vi "9402_UI.vi"(8 "error in (no error)":errorcluster, 11 "Node Ptr":T1 format="%.0x") -> (0 "error out":errorcluster)   [LabVIEW 2020, in "Modules.lvlib" / "9402.lvclass"]
uses:
  9402.lvclass
  <vilib>/NI VeriStand/Custom Device API/Custom Device Item Ref.ctl
  RSI Module/SubPanel Command.ctl
  C:/Users/nitest/Desktop/Git 2020/niveristand-scan-engine-module-libraries/Source/RSI Module/RSI Module.lvclass
  9402.lvclass/9402.ctl
  RSI Module/RSI Module.lvclass
  <vilib>/NI VeriStand/Custom Device API/Custom Device API.lvlib
panel:
  in  "_Channels":u32[](array[ring]) items=["Input", "Output"]
  out "_Selected Channel(s) Settings Label":string="Selected Channel(s) Settings"
  in  "Channels":i32[](listbox)
  in  "LineDirectionVal":u32(ring) caption="Direction" items=["Input", "Output"]
  in  "SubPanel Event":refnum<user-event>
  in  "Header":cluster{"Section Name":string}={"Section Name"="NI 9205 Settings"}
  in  "BadLineDirectionVal":u32(ring) caption="Direction" items=["Input", "Output", "X"]
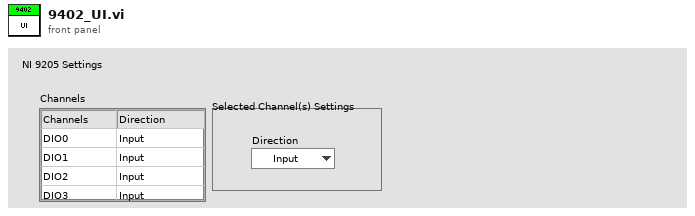
[diagram p1: front panel]
types:
  T1 = typedef "Custom Device API.lvlib/Custom Device Item Ref.ctl" = u64
  T2 = typedef "Modules.lvlib/RSI Module.lvclass/Module Models.ctl" = enum16{"Empty", "NI 9201", "NI 9203", "NI 9205", "NI 9206", "NI 9207", "NI 9208", "NI 9209", "NI 9210", "NI 9211", "NI 9212", "NI 9213", "NI 9214", "NI 9215", "NI 9216", "NI 9217", "NI 9219", "NI 9220", "NI 9221", "NI 9222", "NI 9223", "NI 9224", "NI 9225", "NI 9226", "NI 9227", "NI 9228", "NI 9229", "NI 9233", "NI 9234", "NI 9235", "NI 9236", "NI 9237", "NI 9239", "NI 9242", "NI 9244", "NI 9253", "NI 9263", "NI 9264", "NI 9265", "NI 9266", "NI 9269", "NI 9344", "NI 9350", "NI 9375", "NI 9401", "NI 9402", "NI 9403", "NI 9411", "NI 9421", "NI 9422", "NI 9423", "NI 9425", "NI 9426", "NI 9435", "NI 9436", "NI 9437", "NI 9472", "NI 9474", "NI 9475", "NI 9476", "NI 9477", "NI 9478", "NI 9481", "NI 9482", "NI 9485"}
  T3 = typedef "Modules.lvlib/RSI Module.lvclass/SubPanel Command.ctl" = enum16{"Stop"}
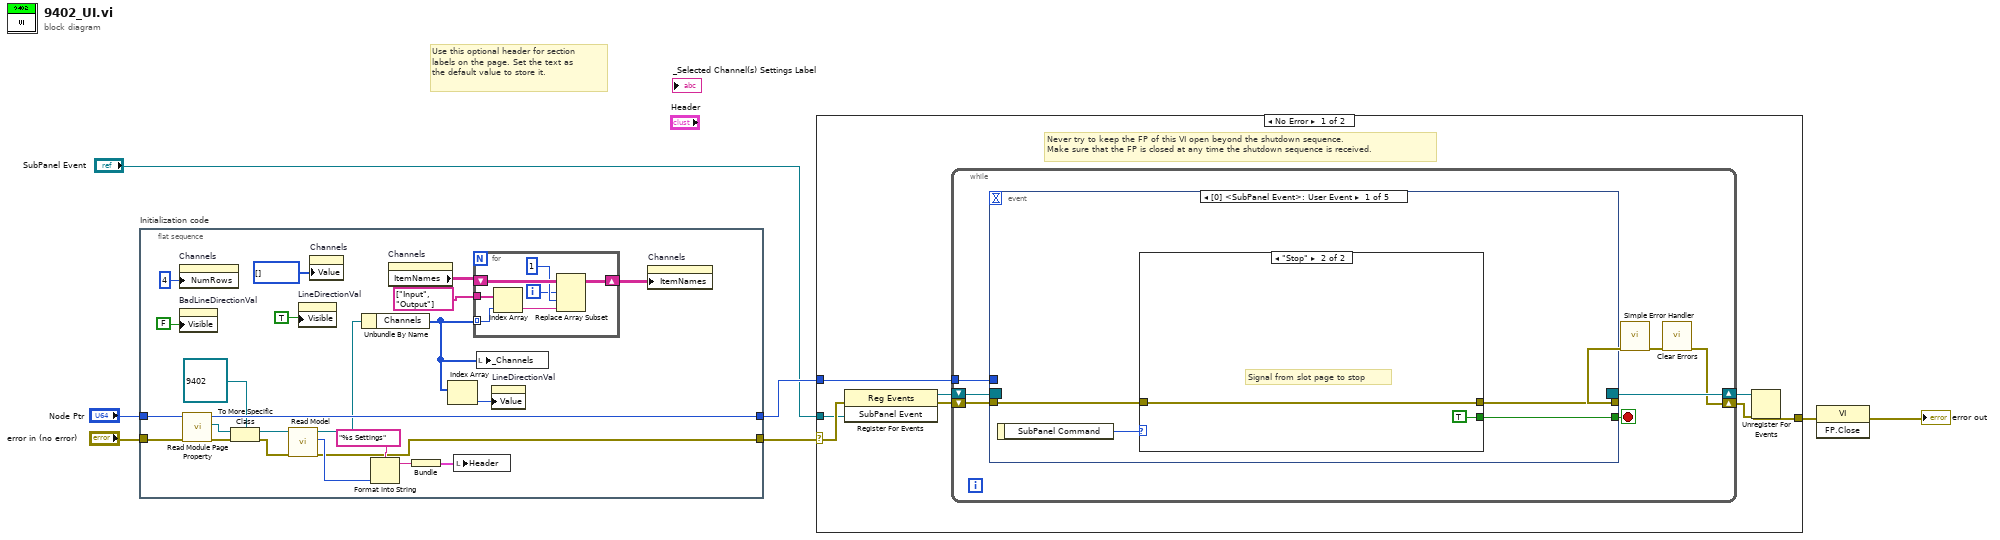
[diagram p0: block diagram]
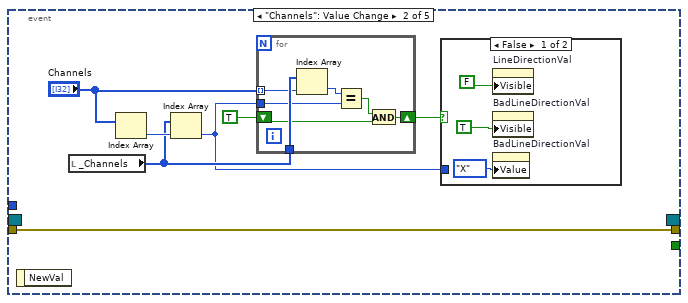
[diagram p3: hidden frame]
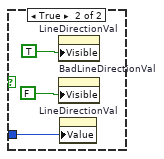
[diagram p4: hidden frame]
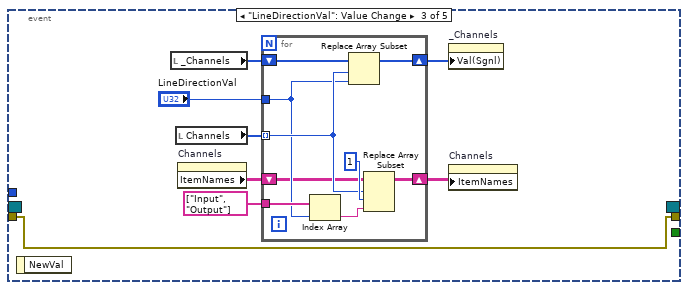
[diagram p5: hidden frame]
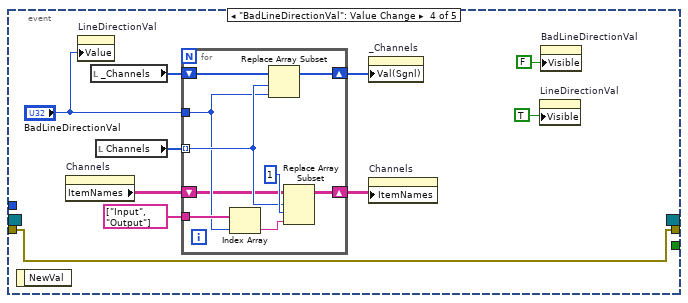
[diagram p6: hidden frame]
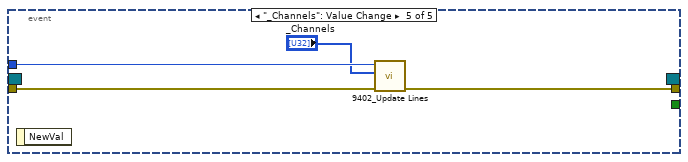
[diagram p7: hidden frame]
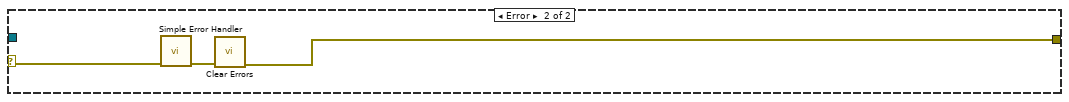
[diagram p8: hidden frame]
diagram:
  # "Use this optional header for section labels on the page. Set the text as the default value to store it."
  n1 = flat-sequence "Initialization code" {
    tunnel: "error in (no error)" -> [w29]
    tunnel: "Node Ptr" -> [w30]
    tunnel: [w17] -> w1
    tunnel: [w28] -> w4
    frame #0 {
      n2 = property on="Channels" class="MCListbox (strict)"("NumRows"=u32 4 ("Number of Rows")) -> ()  [unwired: 2 in, 2 out]
      n3 = property on="BadLineDirectionVal" class="Ring (strict)"("Visible"=FALSE) -> ()  [unwired: 2 in, 2 out]
      n4 = call "Read Module Page Property.vi"("error in (no error)"=w29, "Node Ptr In"=w30) -> ("error out"=w27:errorcluster, "RSI Module"=w25:refnum<class "RSI Module.lvclass">, "Node Ptr Out"=w28:T1)  [unwired: 7 in]
      n5 = To More Specific Class(target class=refnum<class "9402.lvclass"> refnum ("9205 in"), reference=w25, error in=w27) -> (specific class reference=w24:refnum<class "9402.lvclass">, error out=w23:errorcluster)
      n6 = call "Read Model.vi"("error in (no error)"=w23, "RSI Module in"=w24) -> ("error out"=w17:errorcluster, "Model"=w21:T2, "RSI Module out"=w18:refnum<class "9402.lvclass">)  [unwired: 7 in]
      n7 = property on="LineDirectionVal" class="Ring (strict)"("Visible"=TRUE) -> ()  [unwired: 2 in, 2 out]
      n8 = property on="Channels" class="MCListbox (strict)"("Value"=i32[] [] ("Channels")) -> ()  [unwired: 2 in, 2 out]
      n9 = Unbundle By Name(w18) -> ("Channels"=w8:u32[])
      n10 = Format Into String(format string="%s Settings", w21) -> (resulting string=w19:string)  [unwired: 2 in, 1 out]
      n11 = property on="Channels" class="MCListbox (strict)"() -> ("ItemNames"=w12:string[][])  [unwired: 2 in, 2 out]
      n12 = Bundle(w19) -> (w22:cluster{string})  [unwired: 1 in]
      n13 = Index Array(array=w8) -> (element=w9:u32)  [unwired: 1 in]
      n14 = local write "Header"(w22) -> ()
      n15 = for {
        tunnel: w8 -> [w36] mode=indexing
        shift-right: [w35] -> w11
        shift-left: w12 -> [w34]
        tunnel: string[] ["Input", "Output"] -> [w37]
        i -> [w32]
        n16 = Index Array(array=w37, index=w36) -> (element=w31:string)
        n17 = Replace Array Subset(array=w34, new element=w31, index (row)=w32, index (col)=1 ("disabled index (col)")) -> (w35:string[][])
      }
      n18 = local write "_Channels"(w8) -> ()
      n19 = property on="LineDirectionVal" class="Ring (strict)"("Value"=w9) -> ()  [unwired: 2 in, 2 out]
      n20 = property on="Channels" class="MCListbox (strict)"("ItemNames"=w11) -> ()  [unwired: 2 in, 2 out]
    }
  }
  n21 = case shown="No Error" w1 {
    selector: w1 -> [w39 w123]
    tunnel: [w43 w121] -> w7
    tunnel: w4 -> [w40 _]
    tunnel: "SubPanel Event" -> [w38 _]
    frame No Error {
      # "Never try to keep the FP of this VI open beyond the shutdown sequence.\nMake sure that the FP is closed at any time the shutdown sequence is received."
      n22 = register-events(error in=w39, w38) -> (reference out=w41:refnum<event-registration>, error out=w42:errorcluster)  [unwired: 1 in]
      n23 = while {
        tunnel: w40 -> [w49]
        shift-right: [w46] -> w44
        shift-left: w42 -> [w52]
        shift-right: [w53] -> w45
        shift-left: w41 -> [w51]
        stop <- w50 stop-if-true
        n24 = event shown="[0] <SubPanel Event>: User Event" {
          selector: w51 -> [_ _ _ _ _]
          dyn-events: [_ _ _ _ _] -> w53
          timeout: _ -> [_ _ _ _ _]
          tunnel: w52 -> [w56 w63 w81 w101 w119]
          tunnel: [w55 _ _ _ _] -> w50
          tunnel: [w54 w63 w81 w101 w120] -> w48
          tunnel: w49 -> [_ _ _ _ w118]
          event User Event {
            n25 = event-data() -> ("SubPanel Command"=w57:T3)  [unwired: 1 out]
            n26 = case shown="\"Stop\"" w57 {
              tunnel: w56 -> [w58 w59]
              tunnel: [w58 w59] -> w54
              tunnel: [_ TRUE] -> w55
              frame Default {
              }
              frame "Stop" {
                # "Signal from slot page to stop"
              }
            }
          }
          event "Channels": Value Change {
            n27 = event-data() -> ()  [unwired: 2 out]
            n28 = local read "_Channels"() -> (w64:u32[])
            n29 = Index Array(array="Channels") -> (element=w66:i32)  [unwired: 1 in]
            n30 = Index Array(array=w64, index=w66) -> (element=w61:u32)
            n31 = for {
              tunnel: "Channels" -> [w79] mode=indexing
              tunnel: w64 -> [w80]
              tunnel: w61 -> [w77]
              shift-right: [w75] -> w62
              shift-left: TRUE -> [w74]
              n32 = Index Array(array=w80, index=w79) -> (element=w78:u32)
              n33 = Equal?(x=w78, y=w77) -> (x = y?=w76:bool)
              n34 = And(x=w76, y=w74) -> (x .and. y?=w75:bool)
            }
            n35 = case shown="False" w62 {
              tunnel: w61 -> [_ w71]
              frame False {
                n36 = property on="LineDirectionVal" class="Ring (strict)"("Visible"=FALSE) -> ()  [unwired: 2 in, 2 out]
                n37 = property on="BadLineDirectionVal" class="Ring (strict)"("Visible"=TRUE) -> ()  [unwired: 2 in, 2 out]
                n38 = property on="BadLineDirectionVal" class="Ring (strict)"("Value"=enum16{"0", "1", "X"}."X" ("BadNumOutputSyncRegs")) -> ()  [unwired: 2 in, 2 out]
              }
              frame True {
                n39 = property on="LineDirectionVal" class="Ring (strict)"("Visible"=TRUE) -> ()  [unwired: 2 in, 2 out]
                n40 = property on="BadLineDirectionVal" class="Ring (strict)"("Visible"=FALSE) -> ()  [unwired: 2 in, 2 out]
                n41 = property on="LineDirectionVal" class="Ring (strict)"("Value"=w71) -> ()  [unwired: 2 in, 2 out]
              }
            }
          }
          event "LineDirectionVal": Value Change {
            n42 = event-data() -> ()  [unwired: 2 out]
            n43 = local read "_Channels"() -> (w85:u32[])
            n44 = local read "Channels"() -> (w86:i32[])
            n45 = property on="Channels" class="MCListbox (strict)"() -> ("ItemNames"=w83:string[][])  [unwired: 2 in, 2 out]
            n46 = for {
              tunnel: "LineDirectionVal" -> [w91]
              tunnel: w86 -> [w94] mode=indexing
              shift-right: [w96] -> w84
              shift-left: w85 -> [w97]
              tunnel: string[] ["Input", "Output"] -> [w93]
              shift-right: [w89] -> w82
              shift-left: w83 -> [w90]
              n47 = Index Array(array=w93, index=w91) -> (element=w92:string)
              n48 = Replace Array Subset(array=w97, new element=w91, index=w94) -> (w96:u32[])
              n49 = Replace Array Subset(array=w90, new element=w92, index (row)=w94, index (col)=1 ("disabled index (col)")) -> (w89:string[][])
            }
            n50 = property on="_Channels" class="Arr (strict)"("Val(Sgnl)"=w84) -> ()  [unwired: 2 in, 2 out]
            n51 = property on="Channels" class="MCListbox (strict)"("ItemNames"=w82) -> ()  [unwired: 2 in, 2 out]
          }
          event "BadLineDirectionVal": Value Change {
            n52 = event-data() -> ()  [unwired: 2 out]
            n53 = property on="Channels" class="MCListbox (strict)"() -> ("ItemNames"=w103:string[][])  [unwired: 2 in, 2 out]
            n54 = property on="LineDirectionVal" class="Ring (strict)"("Value"="BadLineDirectionVal") -> ()  [unwired: 2 in, 2 out]
            n55 = local read "_Channels"() -> (w105:u32[])
            n56 = local read "Channels"() -> (w106:i32[])
            n57 = for {
              tunnel: "BadLineDirectionVal" -> [w110]
              tunnel: w106 -> [w113] mode=indexing
              shift-right: [w115] -> w104
              shift-left: w105 -> [w116]
              tunnel: string[] ["Input", "Output"] -> [w112]
              shift-right: [w108] -> w102
              shift-left: w103 -> [w109]
              n58 = Index Array(array=w112, index=w110) -> (element=w111:string)
              n59 = Replace Array Subset(array=w116, new element=w110, index=w113) -> (w115:u32[])
              n60 = Replace Array Subset(array=w109, new element=w111, index (row)=w113, index (col)=1 ("disabled index (col)")) -> (w108:string[][])
            }
            n61 = property on="_Channels" class="Arr (strict)"("Val(Sgnl)"=w104) -> ()  [unwired: 2 in, 2 out]
            n62 = property on="Channels" class="MCListbox (strict)"("ItemNames"=w102) -> ()  [unwired: 2 in, 2 out]
            n63 = property on="LineDirectionVal" class="Ring (strict)"("Visible"=TRUE) -> ()  [unwired: 2 in, 2 out]
            n64 = property on="BadLineDirectionVal" class="Ring (strict)"("Visible"=FALSE) -> ()  [unwired: 2 in, 2 out]
          }
          event "_Channels": Value Change {
            n65 = event-data() -> ()  [unwired: 2 out]
            n66 = call "9402_Update Lines.vi"("error in (no error)"=w119, "Line directions"="_Channels", "Node Ptr in"=w118) -> ("error out"=w120:errorcluster)  [unwired: 7 in, 1 out]
          }
        }
        n67 = call <vilib>:"Simple Error Handler.vi"("error in (no error)"=w48) -> ("error out"=w47:errorcluster)  [unwired: 1 in, 7 out]
        n68 = call <vilib>:"Clear Errors.vi"("error in (no error)"=w47) -> ("error out"=w46:errorcluster)  [unwired: 1 in, 5 out]
      }
      n69 = Unregister For Events(event registration refnum=w45, error in=w44) -> (error out=w43:errorcluster)
    }
    frame Error {
      n70 = call <vilib>:"Simple Error Handler.vi"("error in (no error)"=w123) -> ("error out"=w122:errorcluster)  [unwired: 1 in, 7 out]
      n71 = call <vilib>:"Clear Errors.vi"("error in (no error)"=w122) -> ("error out"=w121:errorcluster)  [unwired: 1 in, 5 out]
    }
  }
  n72 = invoke class="VI" method="FP.Close"(error in=w7) -> (error out=→"error out":errorcluster)  [unwired: 2 in, 2 out]
